vi "config_file_accessor.vi"(1 "Configuration In":T1={"Alkalinity Calculation Functions"={"HCl Temp Correction Function"="", "Sample Temp Correction Function"="", "Dosimat Correction Function"="", "Cell Temp Correction Function"="", "HCl Density Function"=""}, "Instrument Settings"={"Relay Port"="COM6", "Agilent Port"="COM5", "Dosimat Port"="COM4", "Thermal Coeffients Path"=path ""}, "Titration Settings"={"Hold Time (sec)"=300, "Initial HCl Increment"=0.0, "Target EMF"=0.0, "Agilent Monitoring Refresh Period"=0.0, "Small HCl Increment"=0.0, "Number of Titration Points"=0}, "Other Settings"={"HCl Concentration"=0.0, "HCl Lot ID"=""}, "Electrode Settings"={"Probe ID - Electrode 1 "=0, "Channel - Electrode 1"=0, "Probe ID - Electrode 2"=0, "Channel - Electrode 2"=0}}, 2 "File Path":path, 3 "Action":u8(ring)=1 items=["read", "write"]) -> (0 "Configuration Out":T1={"Alkalinity Calculation Functions"={"HCl Temp Correction Function"="", "Sample Temp Correction Function"="", "Dosimat Correction Function"="", "Cell Temp Correction Function"="", "HCl Density Function"=""}, "Instrument Settings"={"Relay Port"="COM6", "Agilent Port"="COM5", "Dosimat Port"="COM4", "Thermal Coeffients Path"=path ""}, "Titration Settings"={"Hold Time (sec)"=300, "Initial HCl Increment"=0.0, "Target EMF"=0.0, "Agilent Monitoring Refresh Period"=0.0, "Small HCl Increment"=0.0, "Number of Titration Points"=0}, "Other Settings"={"HCl Concentration"=0.0, "HCl Lot ID"=""}, "Electrode Settings"={"Probe ID - Electrode 1 "=0, "Channel - Electrode 1"=0, "Probe ID - Electrode 2"=0, "Channel - Electrode 2"=0}})   [LabVIEW 2010]
doc: "This VI is used for both writing to and reading the configuration file for the Total Alkalinity Tool Application (TATA, for brevity). It is handy for reading the XML configuration file in, and passing along to the front panel of the parent TATA application, as well as for saving modifications to that configuration file and creating a file if one doesn't yet exist (the parent TATA needs one to operate).\n\nThe data file saved to or loaded from must be of XML format and follow the LabVIEW XML schema."
uses:
  <vilib>/Utility/xml.llb/Read From XML File(string).vi
  <vilib>/Utility/xml.llb/Write to XML File(string).vi
panel:
  out "String":string
  # "This control only works when titration is not actively taking place"
  # "This control only works when titration is not actively taking place"
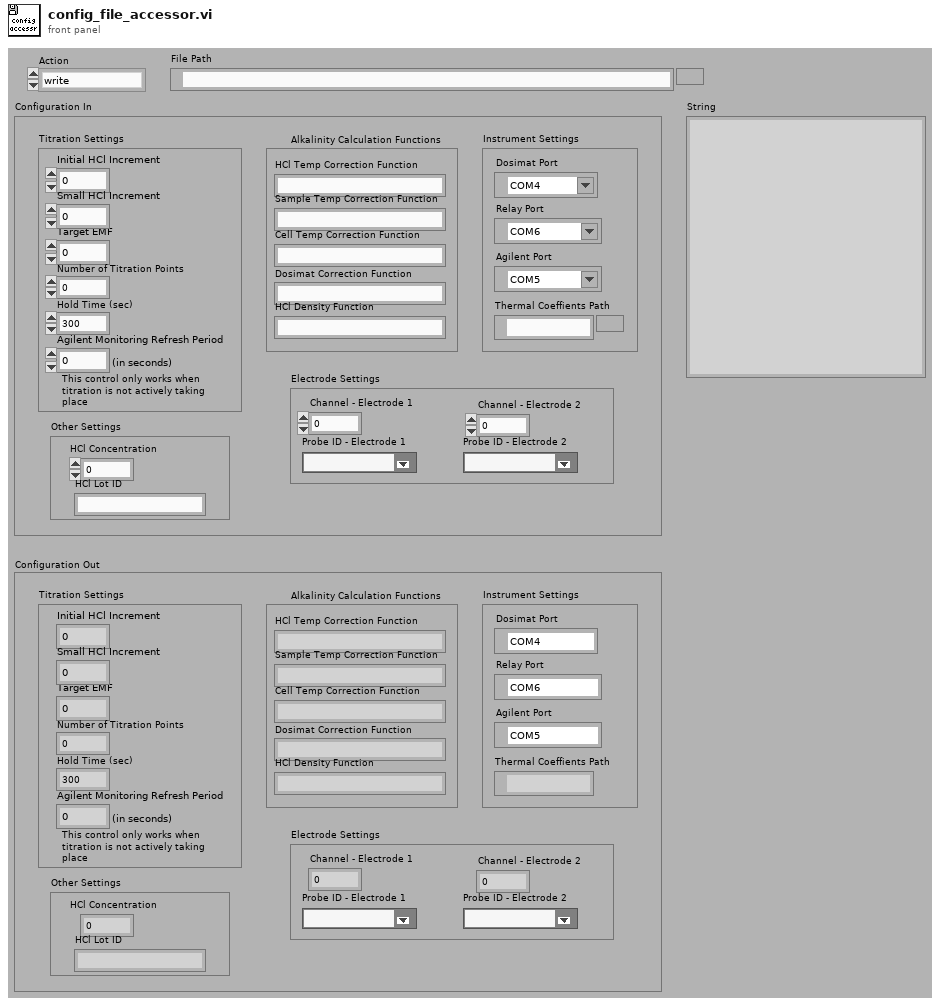
[diagram p1: front panel]
types:
  T1 = cluster{"Alkalinity Calculation Functions":cluster{"HCl Temp Correction Function":string, "Sample Temp Correction Function":string, "Dosimat Correction Function":string, "Cell Temp Correction Function":string, "HCl Density Function":string}, "Instrument Settings":cluster{"Relay Port":refnum<visa-resource-name>, "Agilent Port":refnum<visa-resource-name>, "Dosimat Port":refnum<visa-resource-name>, "Thermal Coeffients Path":path}, "Titration Settings":cluster{"Hold Time (sec)":i16, "Initial HCl Increment":dbl, "Target EMF":dbl, "Agilent Monitoring Refresh Period":dbl, "Small HCl Increment":dbl, "Number of Titration Points":i32}, "Other Settings":cluster{"HCl Concentration":dbl, "HCl Lot ID":string}, "Electrode Settings":cluster{"Probe ID - Electrode 1 ":u16, "Channel - Electrode 1":i32, "Probe ID - Electrode 2":u16, "Channel - Electrode 2":i32}}
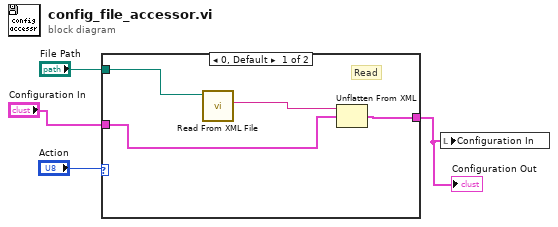
[diagram p0: block diagram]
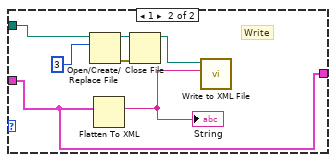
[diagram p2: hidden frame]
diagram:
  n1 = case shown="0, Default" "Action" {
    tunnel: "Configuration In" -> [w6 w9]
    tunnel: "File Path" -> [w7 w10]
    tunnel: [w5 w9] -> w1
    frame 0, Default {
      # "Read"
      n2 = call-poly <vilib>:"Read From XML File.vi"("XML File Path"=w7) -> ("XML Elements"=w8:string)  [unwired: 8 in, 2 out]
      n3 = Unflatten From XML(xml string=w8, type=w6) -> (value=w5:T1)  [unwired: 1 in, 1 out]
    }
    frame 1 {
      # "Write"
      n4 = Open/Create/Replace File(file path (use dialog)=w10, operation (0:open)=3) -> (refnum out=w12:refnum<file>, error out=w11:errorcluster)  [unwired: 4 in, 1 out]
      n5 = Flatten To XML(anything=w9) -> (xml string=w14:string)
      "String" <- w14
      n6 = Close File(refnum=w12, error in=w11) -> (path=w13:path)  [unwired: 1 out]
      n7 = call-poly <vilib>:"Write to XML File.vi"("XML Input"=w14, "XML File Path"=w13) -> ()  [unwired: 7 in, 3 out]
    }
  }
  "Configuration Out" <- w1
  n8 = local write "Configuration In"(w1) -> ()
